vi "Execute Command.vi"(8 "error in (no error)":errorcluster, 10 "command":T2={"Command"=enum."Rx", "Parameters"={"arg1"=0, "arg2"=0}}, 11 "Transceiver Thread in":refnum<class "Transceiver Thread.lvclass">) -> (0 "error out":errorcluster, 2 "state":T1=enum."Start", 3 "Transceiver Thread out":refnum<class "Transceiver Thread.lvclass">)   [LabVIEW 2017, in "DSF Core.lvlib" / "Transceiver Thread.lvclass"]
uses:
  Transceiver Thread.lvclass
  C:/Git/DSF/Core/Classes/Thread/Plugin/Plugin Thread.lvclass
  Interface/Plugin/Command Data.ctl
  Interface/Plugin/Command.ctl
  Interface/Plugin/Command Parameters.ctl
  Interface/Plugin/Response Data.ctl
  Interface/Plugin/Response.ctl
  Interface/Plugin/Response Parameters.ctl
  Interface/Plugin/Plugin Interface.lvclass
  Plugin Thread.lvclass
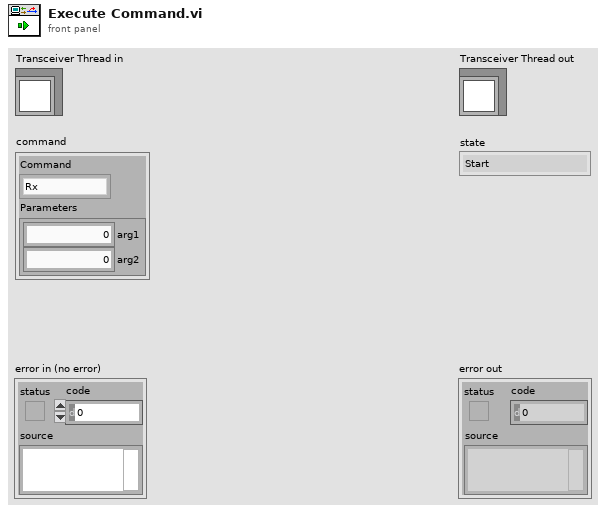
[diagram p1: front panel]
types:
  T1 = typedef "DSF Core.lvlib/Plugin Interface.lvclass/Command.ctl" = enum8{"Idle", "Start", "Set Inline Buffer", "Rx", "Tx", "Shutdown"}
  T2 = typedef "DSF Core.lvlib/Plugin Interface.lvclass/Command Data.ctl" = cluster{"Command":T1, "Parameters":T3}
  T3 = typedef "DSF Core.lvlib/Plugin Interface.lvclass/Command Parameters.ctl" = cluster{"arg1":u64, "arg2":u64}
  T4 = typedef "DSF Core.lvlib/Plugin Interface.lvclass/Response Data.ctl" = cluster{"Response":T5, "Parameters":T6}
  T5 = typedef "DSF Core.lvlib/Plugin Interface.lvclass/Response.ctl" = enum8{"General Ack", "Shutting Down"}
  T6 = typedef "DSF Core.lvlib/Plugin Interface.lvclass/Response Parameters.ctl" = cluster{"arg1":u64, "arg2":u64}
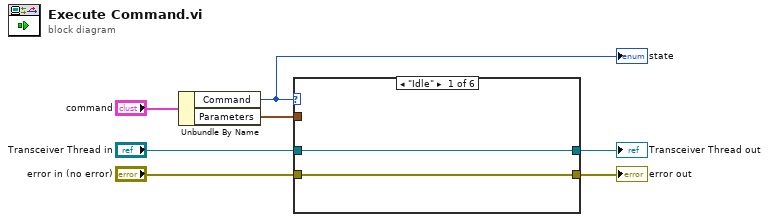
[diagram p0: block diagram]
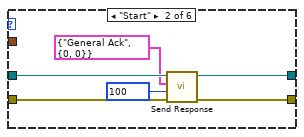
[diagram p2: hidden frame]
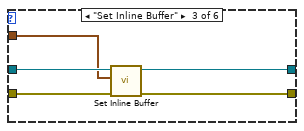
[diagram p3: hidden frame]
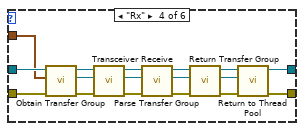
[diagram p4: hidden frame]
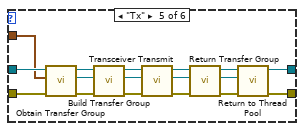
[diagram p5: hidden frame]
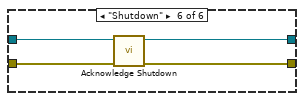
[diagram p6: hidden frame]
diagram:
  n1 = Unbundle By Name("command") -> ("Command"=w1:T1, "Parameters"=w4:T3)
  "state" <- w1
  n2 = case shown="\"Idle\"" w1 {
    tunnel: "Transceiver Thread in" -> [w9 w15 w19 w23 w39 w58]
    tunnel: [w9 w11 w17 w26 w41 w56] -> w3
    tunnel: "error in (no error)" -> [w8 w14 w20 w22 w40 w57]
    tunnel: [w8 w12 w18 w25 w42 w55] -> w2
    tunnel: w4 -> [_ _ w16 w21 w38 _]
    frame "Idle" {
    }
    frame "Start" {
      n3 = call "Send Response.vi"("error in (no error)"=w14, "timeout in ms (0)"=100, "response"=T4 {"Response"=enum."General Ack", "Parameters"={"arg1"=0, "arg2"=0}}, "Plugin Thread in"=w15) -> ("error out"=w12:errorcluster, "Plugin Thread out"=w11:refnum<class "Transceiver Thread.lvclass">)  [unwired: 6 in]
    }
    frame "Set Inline Buffer" {
      n4 = call "Set Inline Buffer.vi"("error in (no error)"=w20, "command parameters"=w16, "Plugin Thread in"=w19) -> ("error out"=w18:errorcluster, "Plugin Thread out"=w17:refnum<class "Transceiver Thread.lvclass">)  [unwired: 7 in]
    }
    frame "Rx" {
      n5 = call "Obtain Transfer Group.vi"("error in (no error)"=w22, "command parameters"=w21, "Transceiver Thread in"=w23) -> ("error out"=w28:errorcluster, "Transfer Group"=w27:refnum<class "Transfer Group.lvclass">, "Transceiver Thread out"=w29:refnum<class "Transceiver Thread.lvclass">)  [unwired: 6 in]
      n6 = call "Transceiver Receive.vi"("error in (no error)"=w28, "Transfer Group in"=w27, "Transceiver Thread in"=w29) -> ("error out"=w36:errorcluster, "Transfer Group out"=w35:refnum<class "Transfer Group.lvclass">, "Transceiver Thread out"=w37:refnum<class "Transceiver Thread.lvclass">)  [unwired: 6 in]
      n7 = call "Parse Transfer Group.vi"("error in (no error)"=w36, "Transfer Group in"=w35, "Plugin Thread in"=w37) -> ("error out"=w33:errorcluster, "Transfer Group out"=w32:refnum<class "Transfer Group.lvclass">, "Plugin Thread out"=w34:refnum<class "Transceiver Thread.lvclass">)  [unwired: 6 in]
      n8 = call "Return Transfer Group.vi"("error in (no error)"=w33, "Transfer Group in"=w32, "Transceiver Thread in"=w34) -> ("error out"=w30:errorcluster, "Transfer Group out"=w24:refnum<class "Transfer Group.lvclass">, "Transceiver Thread out"=w31:refnum<class "Transceiver Thread.lvclass">)  [unwired: 6 in]
      n9 = call "Return to Thread Pool.vi"("error in (no error)"=w30, "Transfer Group in"=w24, "Plugin Thread in"=w31) -> ("error out"=w25:errorcluster, "Plugin Thread out"=w26:refnum<class "Transceiver Thread.lvclass">)  [unwired: 7 in]
    }
    frame "Tx" {
      n10 = call "Obtain Transfer Group.vi"("error in (no error)"=w40, "command parameters"=w38, "Transceiver Thread in"=w39) -> ("error out"=w46:errorcluster, "Transfer Group"=w45:refnum<class "Transfer Group.lvclass">, "Transceiver Thread out"=w47:refnum<class "Transceiver Thread.lvclass">)  [unwired: 6 in]
      n11 = call "Build Transfer Group.vi"("error in (no error)"=w46, "Transfer Group in"=w45, "Plugin Thread in"=w47) -> ("error out"=w53:errorcluster, "Transfer Group out"=w43:refnum<class "Transfer Group.lvclass">, "Plugin Thread out"=w54:refnum<class "Transceiver Thread.lvclass">)  [unwired: 6 in]
      n12 = call "Transceiver Transmit.vi"("error in (no error)"=w53, "Transfer Group in"=w43, "Transceiver Thread in"=w54) -> ("error out"=w51:errorcluster, "Transfer Group out"=w50:refnum<class "Transfer Group.lvclass">, "Transceiver Thread out"=w52:refnum<class "Transceiver Thread.lvclass">)  [unwired: 6 in]
      n13 = call "Return Transfer Group.vi"("error in (no error)"=w51, "Transfer Group in"=w50, "Transceiver Thread in"=w52) -> ("error out"=w48:errorcluster, "Transfer Group out"=w44:refnum<class "Transfer Group.lvclass">, "Transceiver Thread out"=w49:refnum<class "Transceiver Thread.lvclass">)  [unwired: 6 in]
      n14 = call "Return to Thread Pool.vi"("error in (no error)"=w48, "Transfer Group in"=w44, "Plugin Thread in"=w49) -> ("error out"=w42:errorcluster, "Plugin Thread out"=w41:refnum<class "Transceiver Thread.lvclass">)  [unwired: 7 in]
    }
    frame "Shutdown" {
      n15 = call "Acknowledge Shutdown.vi"("error in (no error)"=w57, "Plugin Thread in"=w58) -> ("error out"=w55:errorcluster, "Plugin Thread out"=w56:refnum<class "Transceiver Thread.lvclass">)  [unwired: 8 in]
    }
  }
  "error out" <- w2
  "Transceiver Thread out" <- w3
